vi "ActionVIOnCompile.vi"(8 "error in (no error)":errorcluster, 11 "Device Item Ref in":T1 format="%.0x") -> (0 "error out":errorcluster)   [LabVIEW 2019, in "MD4Logger System Explorer.lvlib"]
uses:
  MD4Logger System Explorer.lvlib
  <vilib>/NI VeriStand/Custom Device API/Custom Device Item Ref.ctl
  Shared/Constants.vi
  <vilib>/NI VeriStand/Custom Device Tools/Custom Device Utility Library/NI VeriStand - Search for Item by Name.vi
  <vilib>/NI VeriStand/Custom Device API/Set Item Property (Variant).vi
  <vilib>/NI VeriStand/Custom Device Tools/Custom Device Utility Library/Custom Device Utility Library.lvlib
  <vilib>/NI VeriStand/Custom Device API/Custom Device API.lvlib
  <vilib>/NI/NIVS Inline Async API/_Data Access System Explorer/Data Access System Explorer.lvlib
  Shared/MD4Logger Shared.lvlib
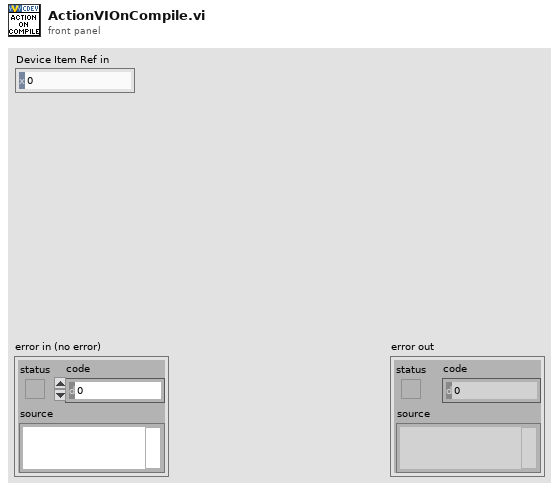
[diagram p1: front panel]
types:
  T1 = typedef "Custom Device API.lvlib/Custom Device Item Ref.ctl" = u64
  T2 = cluster{"Name":string, "Type":enum16{"Output/Write", "Input/Read", "Input/ReadWrite"}, "VS Refs":T1[]}
  T3 = enum16{"Output/Write", "Input/Read", "Input/ReadWrite"}
  T4 = typedef "Custom Device API.lvlib/Custom Device Item Info.ctl" = cluster{"Name":string, "Is Channel":bool, "GUID":string, "Is Waveform":bool}
  T5 = cluster{"Name":string, "Type":enum16{"Output/Write", "Input/Read", "Input/ReadWrite"}, "VS Refs":T1[]}[]
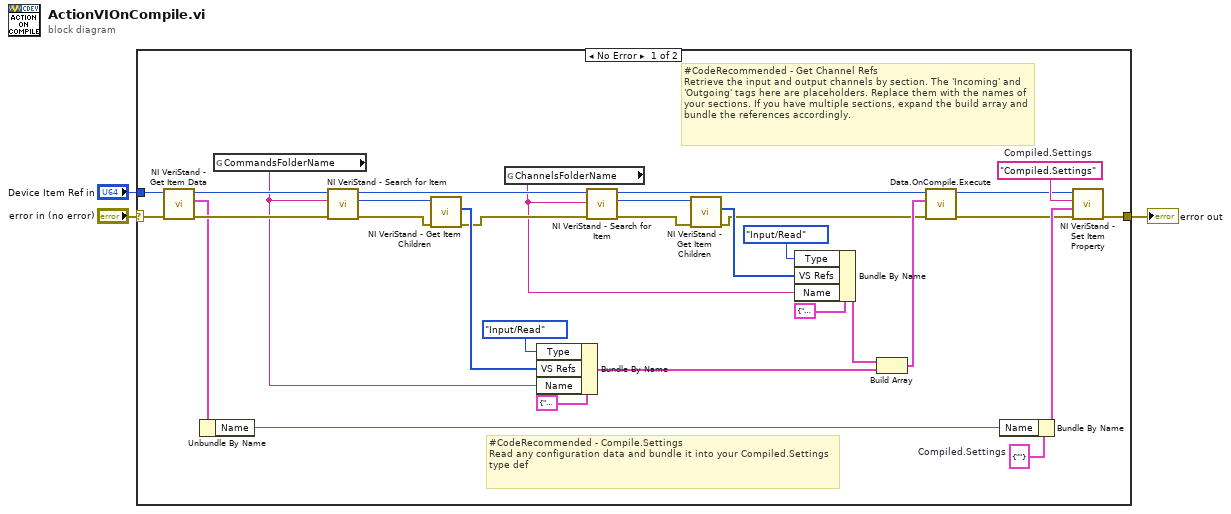
[diagram p0: block diagram]
diagram:
  n1 = case shown="No Error" "error in (no error)" {
    selector: "error in (no error)" -> [w28 w35]
    tunnel: [w29 w35] -> w2
    tunnel: "Device Item Ref in" -> [w27 _]
    frame No Error {
      w7 = cluster{"Name":string} {"Name"=""}  # Compiled.Settings
      w31 = "Compiled.Settings"  # Compiled.Settings
      # "#CodeRecommended - Get Channel Refs\nRetrieve the input and output channels by section. The 'Incoming' and 'Outgoing' tags here are placeholders. Replace them with the names of your sections. If you have multiple sections, expand the build array and bundle the references accordingly."
      # "#CodeRecommended - Compile.Settings\nRead any configuration data and bundle it into your Compiled.Settings type def"
      n2 = call <vilib>:"NI VeriStand - Get Item Data.vi"("error in (no error)"=w28, "Item Ref in"=w27) -> ("error out"=w25:errorcluster, "Item Info"=w24:T4, "Item Ref out"=w26:T1)  [unwired: 6 in, 1 out]
      n3 = Unbundle By Name(w24) -> ("Name"=w23:string)
      n4 = global read "Constants.vi" "CommandsFolderName"() -> (w4:string)
      n5 = call-poly <vilib>:"NI VeriStand - Search for Item.vi"("error in"=w25, "Item Name"=w4, "Section Ref in"=w26) -> ("error out"=w34:errorcluster, "Item Ref"=w33:T1, "Section Ref out"=w11:T1)  [unwired: 5 in, 1 out]
      n6 = call <vilib>:"NI VeriStand - Get Item Children.vi"("error in (no error)"=w34, "Item Ref in"=w33) -> ("error out"=w10:errorcluster, "Child Refs"=w22:T1[])  [unwired: 6 in, 2 out]
      n7 = global read "Constants.vi" "ChannelsFolderName"() -> (w5:string)
      n8 = Bundle By Name(cluster=T2 {"Name"="", "Type"=enum."Output/Write", "VS Refs"=[]} ("Group"), "Type"=T3."Input/Read", "VS Refs"=w22, "Name"=w4) -> (w14:T2)
      n9 = call-poly <vilib>:"NI VeriStand - Search for Item.vi"("error in"=w10, "Item Name"=w5, "Section Ref in"=w11) -> ("error out"=w32:errorcluster, "Item Ref"=w6:T1, "Section Ref out"=w12:T1)  [unwired: 5 in, 1 out]
      n10 = call <vilib>:"NI VeriStand - Get Item Children.vi"("error in (no error)"=w32, "Item Ref in"=w6) -> ("error out"=w13:errorcluster, "Child Refs"=w18:T1[])  [unwired: 6 in, 2 out]
      n11 = Bundle By Name(cluster=T2 {"Name"="", "Type"=enum."Output/Write", "VS Refs"=[]} ("Group"), "Type"=T3."Input/Read", "VS Refs"=w18, "Name"=w5) -> (w20:T2)
      n12 = Build Array(w20, w14) -> (w17:T5)
      n13 = call <vilib>:"Data.OnCompile.Execute.vi"("error in"=w13, "VS Ref Groups"=w17, "Custom Device Ref"=w12) -> ("error out"=w9:errorcluster, "Custom Device Ref"=w8:T1)  [unwired: 7 in]
      n14 = Bundle By Name(cluster=w7, "Name"=w23) -> (w30:cluster{"Name":string})
      n15 = call-poly <vilib>:"NI VeriStand - Set Item Property.vi"("error in (no error)"=w9, "Value"=w30, "Property Name"=w31, "Item Ref in"=w8) -> ("error out"=w29:errorcluster)  [unwired: 5 in, 2 out]
    }
    frame Error {
    }
  }
  "error out" <- w2
